vi "Get VISA资源名称.vi"(11 "THM-V6数字型温湿度 in":refnum<class "THM-V6数字型温湿度.lvclass">) -> (2 "VISA资源名称":refnum<visa-resource-name>, 3 "THM-V6数字型温湿度 out":refnum<class "THM-V6数字型温湿度.lvclass">)   [LabVIEW 2016, in "THM-V6数字型温湿度.lvlib" / "THM-V6数字型温湿度.lvclass"]
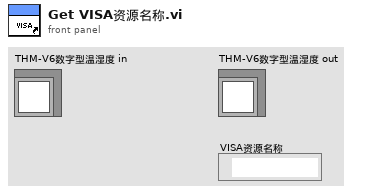
[diagram p1: front panel]
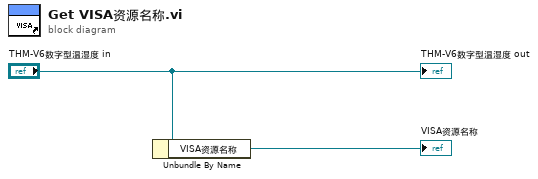
[diagram p0: block diagram]
diagram:
  n1 = Unbundle By Name("THM-V6数字型温湿度 in") -> ("VISA资源名称"=→"VISA资源名称":refnum<visa-resource-name>)
  "THM-V6数字型温湿度 out" <- "THM-V6数字型温湿度 in"
